vi "ApplyQueuedMapUpdates.vi"(8 "error in (no error)":errorcluster, 11 "OccupancyGridWorldMap in":refnum<class "NI_Robotics_OccupancyGridWorldMap.lvclass">) -> (0 "error out":errorcluster, 3 "OccupancyGridWorldMap out":refnum<class "NI_Robotics_OccupancyGridWorldMap.lvclass">)   [LabVIEW 2017, in "NI_Robotics_OccupancyGridWorldMap.lvclass"]
uses:
  <vilib>/robotics/Navigation/shared/WorldMap/OccupancyGridWorldMap/NI_Robotics_OccupancyGridWorldMap.lvclass
  <vilib>/robotics/Navigation/shared/WorldMap/OccupancyGridWorldMap/NI_Robotics_OccupancyGridWorldMap.lvclass/NI_Robotics_OccupancyGridWorldMap.ctl
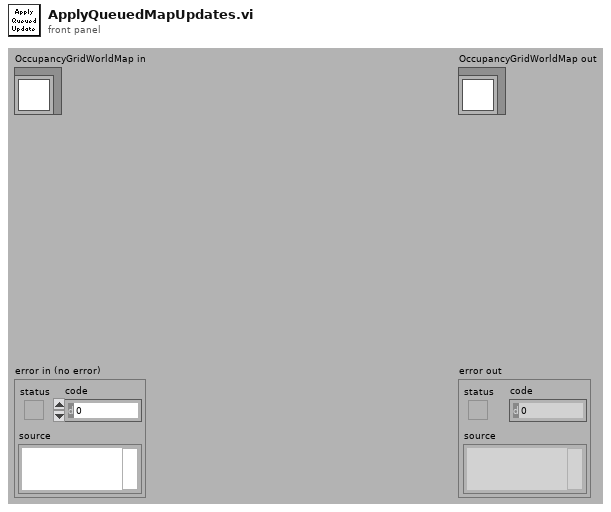
[diagram p1: front panel]
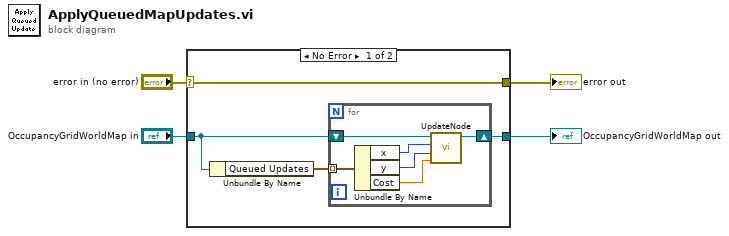
[diagram p0: block diagram]
diagram:
  n1 = case shown="No Error" "error in (no error)" {
    selector: "error in (no error)" -> [w5 w15]
    tunnel: "OccupancyGridWorldMap in" -> [w7 w16]
    tunnel: [w6 w16] -> w3
    tunnel: [w5 w15] -> w1
    frame No Error {
      n2 = Unbundle By Name(w7) -> ("Queued Updates"=w8:cluster{"x":i32, "y":i32, "Cost":dbl}[])
      n3 = for {
        tunnel: w8 -> [w14] mode=indexing
        shift-right: [w9] -> w6
        shift-left: w7 -> [w13]
        n4 = Unbundle By Name(w14) -> ("x"=w12:i32, "y"=w11:i32, "Cost"=w10:dbl)
        n5 = call-dynamic "UpdateNode.vi"("Cost"=w10, "y"=w11, "x"=w12, "OccupancyGridWorldMap in"=w13) -> ("OccupancyGridWorldMap out"=w9:refnum<class "NI_Robotics_OccupancyGridWorldMap.lvclass">)  [unwired: 7 in]
      }
    }
    frame Error {
    }
  }
  "error out" <- w1
  "OccupancyGridWorldMap out" <- w3
